vi "Set-Point Enforcement Waveforms.vi"() -> (0 "Output Waveforms":waveform(dbl)[](array[waveform]))   [LabVIEW 2013]
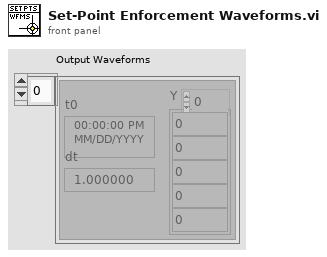
[diagram p1: front panel]
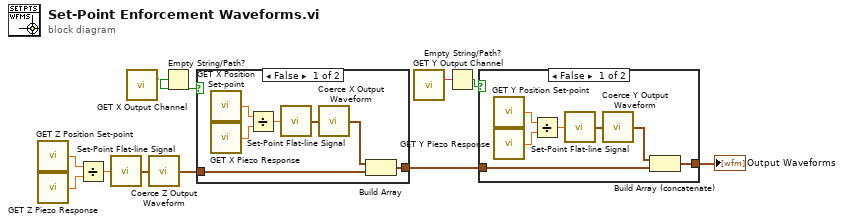
[diagram p0: block diagram]
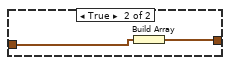
[diagram p3: hidden frame]
diagram:
  n1 = call "GET Z Position Set-point.vi"() -> ("Z Position Set-point"=w7:dbl)
  n2 = call "GET Z Piezo Response.vi"() -> ("Z Piezo Response"=w8:dbl)
  n3 = Divide(x=w7, y=w8) -> (x/y=w9:dbl)
  n4 = call "Set-Point Flat-line Signal.vi"("Flatline Offset"=w9) -> ("Flatline Signal"=w2:waveform(dbl))
  n5 = call "GET X Output Channel.vi"() -> ("X Output Channel"=w5:string)
  n6 = call "Coerce Z Output Waveform.vi"("X Output Waveform"=w2) -> ("Coerced X Output Waveform"=w1:waveform(dbl))
  n7 = Empty String/Path?(string/path=w5) -> (empty?=w6:bool)
  n8 = case shown="False" w6 {
    tunnel: w1 -> [w15 w19]
    tunnel: [w14 w20] -> w10
    frame False {
      n9 = call "GET X Position Set-point.vi"() -> ("X Position Set-point"=w17:dbl)
      n10 = call "GET X Piezo Response.vi"() -> ("X Piezo Response"=w18:dbl)
      n11 = Divide(x=w17, y=w18) -> (x/y=w16:dbl)
      n12 = call "Set-Point Flat-line Signal.vi"("Flatline Offset"=w16) -> ("Flatline Signal"=w13:waveform(dbl))
      n13 = call "Coerce X Output Waveform.vi"("X Output Waveform"=w13) -> ("Coerced X Output Waveform"=w12:waveform(dbl))
      n14 = Build Array(w12, w15) -> (w14:waveform(dbl)[])
    }
    frame True {
      n15 = Build Array(w19) -> (w20:waveform(dbl)[])
    }
  }
  n16 = call "GET Y Output Channel.vi"() -> ("Y Output Channel"=w3:string)
  n17 = Empty String/Path?(string/path=w3) -> (empty?=w4:bool)
  n18 = case shown="False" w4 {
    tunnel: w10 -> [w24 w28]
    tunnel: [w23 w28] -> w11
    frame False {
      n19 = call "GET Y Position Set-point.vi"() -> ("Y Position Set-point"=w26:dbl)
      n20 = call "GET Y Piezo Response.vi"() -> ("Y Piezo Response"=w27:dbl)
      n21 = Divide(x=w26, y=w27) -> (x/y=w25:dbl)
      n22 = call "Set-Point Flat-line Signal.vi"("Flatline Offset"=w25) -> ("Flatline Signal"=w22:waveform(dbl))
      n23 = call "Coerce Y Output Waveform.vi"("X Output Waveform"=w22) -> ("Coerced X Output Waveform"=w21:waveform(dbl))
      n24 = Build Array (concatenate)(w21, w24) -> (w23:waveform(dbl)[])
    }
    frame True {
    }
  }
  "Output Waveforms" <- w11
